vi "refs_get.vi"(8 "error in":errorcluster) -> (0 "error out":errorcluster, 1 "stat 3 ref":refnum<vi>, 2 "stat 2 ref":refnum<vi>, 3 "stat 1 ref":refnum<vi>, 4 "error ref":refnum<vi>, 5 "btn stop ref":refnum<vi>, 6 "skip ref":refnum<vi>)   [LabVIEW 2013]
uses:
  refs_var.vi
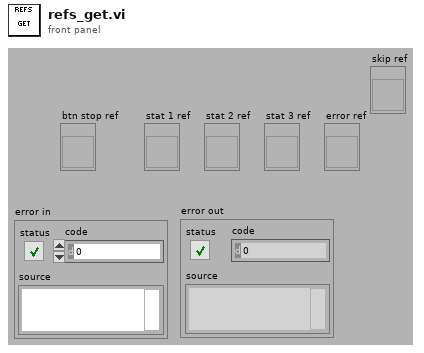
[diagram p1: front panel]
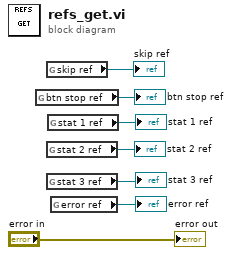
[diagram p0: block diagram]
diagram:
  n1 = global read "refs_var.vi" "btn stop ref"() -> (→"btn stop ref":refnum<vi>)
  n2 = global read "refs_var.vi" "skip ref"() -> (→"skip ref":refnum<vi>)
  n3 = global read "refs_var.vi" "stat 2 ref"() -> (→"stat 2 ref":refnum<vi>)
  n4 = global read "refs_var.vi" "stat 3 ref"() -> (→"stat 3 ref":refnum<vi>)
  n5 = global read "refs_var.vi" "stat 1 ref"() -> (→"stat 1 ref":refnum<vi>)
  n6 = global read "refs_var.vi" "error ref"() -> (→"error ref":refnum<vi>)
  "error out" <- "error in"
